vi "Move.vi"(7 "VI":refnum<vi>, 8 "Error":errorcluster, 11 "(FPPos)":refnum<class "(FPPos).lvclass">) -> (0 "Error Out":errorcluster, 3 "(FPPos) Out":refnum<class "(FPPos).lvclass">, 5 "VI Out":refnum<vi>)   [LabVIEW 2016, in "(FPPos).lvclass"]
uses:
  (FPPos).lvclass
  TypeDefs_Utility/ENUM RB_Pos_Quadrant Position.ctl
  TypeDefs_Utility/Cluster_Pos_Top Left position.ctl
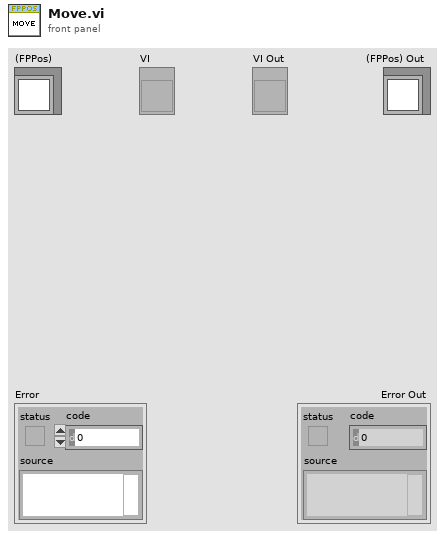
[diagram p1: front panel]
types:
  T1 = typedef "Cluster_Pos_Top Left position.ctl" = cluster{"Left":i16, "Top":i16}
  T2 = typedef "ENUM RB_Pos_Quadrant Position.ctl" = enum32{"LFT-TOP", "MID-TOP", "RGT-TOP", "LFT-CTR", "MID-CTR", "RGT-CTR", "LFT-BOT", "MID-BOT", "RGT-BOT"}
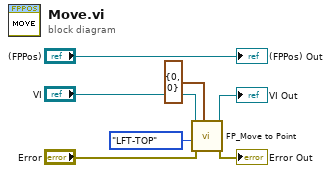
[diagram p0: block diagram]
diagram:
  n1 = call "FP_Move to Point.vi"("Target Point"=T1 {"Left"=0, "Top"=0}, "Error"="Error", "FP Position"=ENUM_RB_Pos_Quadrant_Position."LFT-TOP", "VI"="VI") -> ("Error Out"=→"Error Out":errorcluster, "VI Out"=→"VI Out":refnum<vi>)  [unwired: 6 in]
  "(FPPos) Out" <- "(FPPos)"
